vi "SailBoatSpeedCalc.vi"(1 "Boat Direction":dbl, 2 "Wind Direction (Rad global coordinates)":dbl, 3 "Wind Speed":dbl, 4 "Velocity Desired In":dbl) -> (0 "Boat Velocity Out":dbl)   [LabVIEW 2012]
doc: "This VI calculates boat speed based on wind speed"
uses:
  <vilib>/Math Plots/2D Math Plots/2D Compass/2D Compass XCtrl/2D Compass.xctl
  <vilib>/Math Plots/2D Math Plots/2D Compass/2D Compass Datatype/Public/Plot Helper (Vector).vi
  <vilib>/Math Plots/2D Math Plots/2D Compass/2D Compass Datatype/2D Compass Datatype.lvclass
panel:
  out "Rel Angle":dbl
  out "Speed Array":dbl[](array[numeric])
  out "Boat Speed wrt Wind Vector":refnum<class "2D Plot Datatype.lvclass">[](xcontrol) caption="2D Compass"
  # "All Directions in Radians"
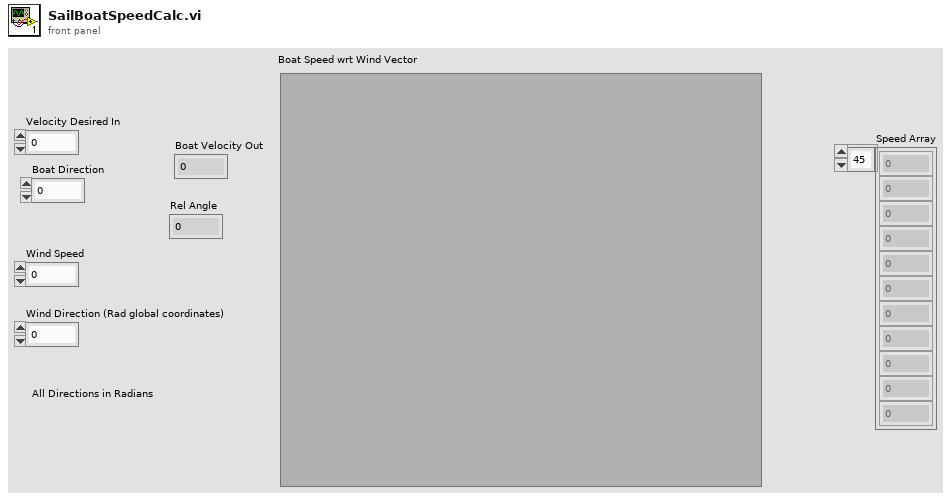
[diagram p1: front panel]
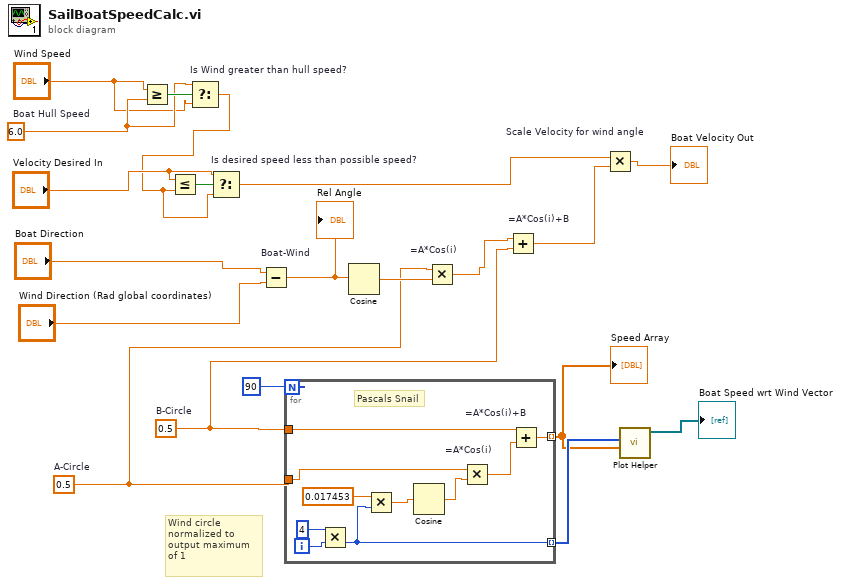
[diagram p0: block diagram]
diagram:
  w11 = 0.5  # B-Circle
  w12 = 0.5  # A-Circle
  w7 = 6.0  # Boat Hull Speed
  # "Wind circle\nnormalized to\noutput maximum\nof 1"
  n1 = Greater Or Equal?(x="Wind Speed", y=w7) -> (x >= y?=w8:bool)
  n2 = Select "Is Wind greater than hull speed?"(t=w7, s=w8, f="Wind Speed") -> (s? t:f=w3:dbl)
  n3 = Less Or Equal?(x="Velocity Desired In", y=w3) -> (x <= y?=w5:bool)
  n4 = Select "Is desired speed less than possible speed?"(t="Velocity Desired In", s=w5, f=w3) -> (s? t:f=w1:dbl)
  n5 = Subtract "Boat-Wind"(x="Boat Direction", y="Wind Direction (Rad global coordinates)") -> (x-y=w14:dbl)
  "Rel Angle" <- w14
  n6 = for {
    N: 90 -> [_]
    tunnel: w12 -> [w30]
    tunnel: w11 -> [w28]
    tunnel: [w27] -> w17 mode=indexing
    tunnel: [w22] -> w18 mode=indexing
    i -> [w24]
    # "Pascals Snail"
    n7 = Multiply(x=4, y=w24) -> (x*y=w22:i32)
    n8 = Multiply(x=0.017453 ("y"), y=w22) -> (x*y=w25:dbl)
    n9 = Cosine(x=w25) -> (cos(x)=w26:dbl)
    n10 = Multiply "=A*Cos(i)"(x=w30, y=w26) -> (x*y=w29:dbl)
    n11 = Add "=A*Cos(i)+B"(x=w28, y=w29) -> (x+y=w27:dbl)
  }
  "Speed Array" <- w17
  n12 = Cosine(x=w14) -> (cos(x)=w13:dbl)
  n13 = Multiply "=A*Cos(i)"(x=w12, y=w13) -> (x*y=w10:dbl)
  n14 = Add "=A*Cos(i)+B"(x=w10, y=w11) -> (x+y=w9:dbl)
  n15 = Multiply "Scale Velocity for wind angle"(x=w1, y=w9) -> (x*y=→"Boat Velocity Out":dbl)
  n16 = call-poly <vilib>:"Plot Helper.vi"("radius vector"=w17, "theta vector"=w18) -> ("2D Plot Class Obj Array out"=→"Boat Speed wrt Wind Vector":refnum<class "2D Plot Datatype.lvclass">[])  [unwired: 2 in, 7 out]
